vi "Elevator Inline PID.vi"(8 "Manual?":bool, 9 "Setpoint":dbl, 10 "Reset":bool, 11 "Cluster":T10={"Setpoint"=0.0, "Output"=0.0, "DriveMotor"={"DeviceStatus"={"status"=FALSE, "code"=0, "source"=""}, "Type"=enum."PWM", "PWM"={"PWM Channel"=enum."Invalid", "DeadBand"={"Name"="", "maxPositivePwm"=0, "minPositivePwm"=0, "centerPwm"=0, "maxNegativePwm"=0, "minNegativePwm"=0, "angularRange"=0}}, "CAN"={"Device Number"=0, "SetOutput VI Ref"=variant(enum8{"Percent VBus", "Current", "Speed", "Position", "Voltage"} enum."Percent VBus"), "GetOutput VI Ref"=variant(refnum<k1> refnum), "Enable VI Ref"=variant(dbl 12.0), "Disable VI Ref"=variant(enum8{"Percent VBus", "Speed", "Position", "Slave", "Unchanged / Invalid"} enum."Percent VBus"), "Data"=variant(enum16{"Controller 1"} enum."Controller 1")}, "Invert"=FALSE, "DIO PWM"={"PWM \"Enable\" Channel"=enum."Invalid", "DIOChannel"=enum."Invalid", "PWM Rate"=0.0}}, "Encoder"={"DevStatus"={"status"=FALSE, "code"=0, "source"=""}, "EncoderIndex"=enum."Invalid", "CounterIndex"=enum."Invalid", "DistancePerCount"=1.0, "Decoding Type"=enum."4x"}, "notifier"=refnum}) -> (3 "Cluster 2":T10={"Setpoint"=0.0, "Output"=0.0, "DriveMotor"={"DeviceStatus"={"status"=FALSE, "code"=0, "source"=""}, "Type"=enum."PWM", "PWM"={"PWM Channel"=enum."Invalid", "DeadBand"={"Name"="", "maxPositivePwm"=0, "minPositivePwm"=0, "centerPwm"=0, "maxNegativePwm"=0, "minNegativePwm"=0, "angularRange"=0}}, "CAN"={"Device Number"=0, "SetOutput VI Ref"=variant(enum8{"Percent VBus", "Current", "Speed", "Position", "Voltage"} enum."Percent VBus"), "GetOutput VI Ref"=variant(refnum<k1> refnum), "Enable VI Ref"=variant(dbl 12.0), "Disable VI Ref"=variant(enum8{"Percent VBus", "Speed", "Position", "Slave", "Unchanged / Invalid"} enum."Percent VBus"), "Data"=variant(enum16{"Controller 1"} enum."Controller 1")}, "Invert"=FALSE, "DIO PWM"={"PWM \"Enable\" Channel"=enum."Invalid", "DIOChannel"=enum."Invalid", "PWM Rate"=0.0}}, "Encoder"={"DevStatus"={"status"=FALSE, "code"=0, "source"=""}, "EncoderIndex"=enum."Invalid", "CounterIndex"=enum."Invalid", "DistancePerCount"=1.0, "Decoding Type"=enum."4x"}, "notifier"=refnum})   [LabVIEW 2017]
uses:
  <vilib>/Rock Robotics/WPI/MotorControl/WPI_MotorControlDeviceRef.ctl
  <vilib>/Rock Robotics/WPI/MotorControl/WPI_MotorControlType.ctl
  <vilib>/Rock Robotics/SystemInterfaces/DIO/FPGA_DIOPWMChannel.ctl
  <vilib>/Rock Robotics/WPI/PWM/WPI_PWMDeadband.ctl
  <vilib>/Rock Robotics/SystemInterfaces/DIO/FPGA_DIOChannel.ctl
  <vilib>/Rock Robotics/WPI/Encoder/WPI_EncoderDevRef.ctl
  <vilib>/Rock Robotics/SystemInterfaces/Encoder/FPGA_EncoderIdx.ctl
  <vilib>/Rock Robotics/SystemInterfaces/Counter/FPGA_CounterCtrSystemIndex.ctl
  <vilib>/Rock Robotics/WPI/Encoder/WPI_EncoderType.ctl
  Typedef/Controller Message.ctl
  Typedef/FGVAction.ctl
  SimulatorVIs/Simulation Input Global.vi
  <vilib>/ptbypt/NI_PtbyPt.lvlib
panel:
  in  "homing speed":dbl=0.05 format="%#_13g"
  in  "min speed":dbl=0.05 format="%#_13g"
  in  "gravity":dbl=0.003 format="%#_13g"
  in  "PIDF gains":cluster{"Kp":dbl, "Ki":dbl, "Kd":dbl, "Kf":dbl}={"Kp"=0.01, "Ki"=0.0, "Kd"=0.06, "Kf"=0.0} {"Kf" format="%.5f"; "Kd" format="%.3f"; "Ki" format="%.3f"; "Kp" format="%.3f"}
  out "Plant Input":dbl(graph)=0.12000000000000001
  in  "output range":cluster{"output high":dbl, "output low":dbl}={"output high"=1.0, "output low"=-1.0} {"output low" format="%.2f"; "output high" format="%.2f"}
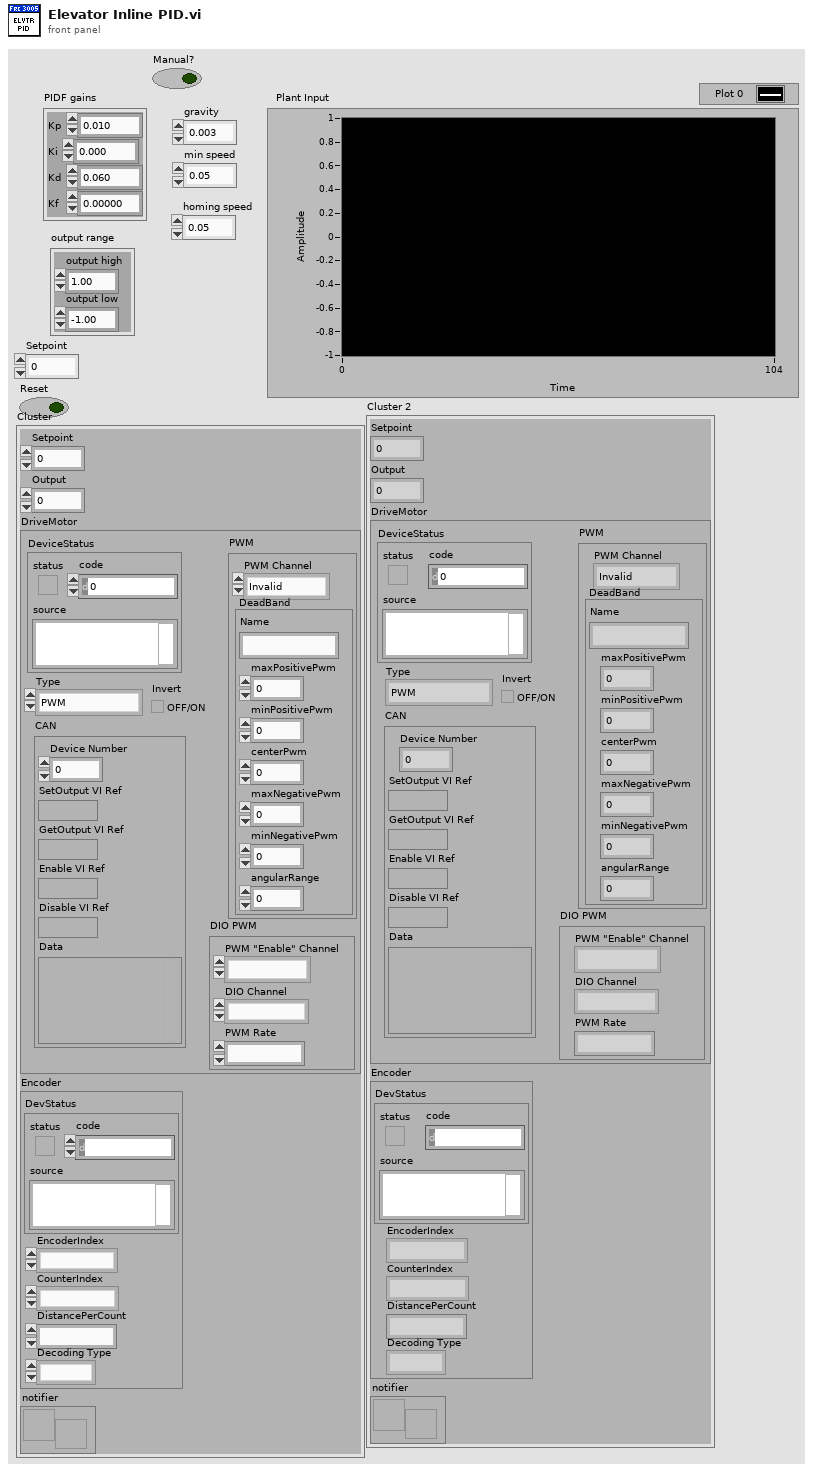
[diagram p1: front panel]
types:
  T1 = typedef "WPI_MotorControlDeviceRef.ctl" = cluster{"DeviceStatus":errorcluster, "Type":T2, "PWM":cluster{"PWM Channel":T3, "DeadBand":T4}, "CAN":cluster{"Device Number":u8, "SetOutput VI Ref":variant, "GetOutput VI Ref":variant, "Enable VI Ref":variant, "Disable VI Ref":variant, "Data":variant}, "Invert":bool, "DIO PWM":cluster{"PWM \"Enable\" Channel":T3, "DIOChannel":T5, "PWM Rate":dbl}}
  T2 = typedef "WPI_MotorControlType.ctl" = enum16{"PWM", "CAN", "DIO PWM"}
  T3 = typedef "FPGA_DIOPWMChannel.ctl" = enum8{"PWM 0", "PWM 1", "PWM 2", "PWM 3", "PWM 4", "PWM 5", "PWM 6", "PWM 7", "PWM 8", "PWM 9", "PWM MXP 0", "PWM MXP 1", "PWM MXP 2", "PWM MXP 3", "PWM MXP 4", "PWM MXP 5", "PWM MXP 6", "PWM MXP 7", "PWM MXP 8", "PWM MXP 9", "Invalid"}
  T4 = typedef "WPI_PWMDeadband.ctl" = cluster{"Name":string, "maxPositivePwm":i32, "minPositivePwm":i32, "centerPwm":i32, "maxNegativePwm":i32, "minNegativePwm":i32, "angularRange":u16}
  T5 = typedef "FPGA_DIOChannel.ctl" = enum8{"DIO 0", "DIO 1", "DIO 2", "DIO 3", "DIO 4", "DIO 5", "DIO 6", "DIO 7", "DIO 8", "DIO 9", "DIO MXP 0", "DIO MXP 1", "DIO MXP 2", "DIO MXP 3", "DIO MXP 4", "DIO MXP 5", "DIO MXP 6", "DIO MXP 7", "DIO MXP 8", "DIO MXP 9", "DIO MXP 10", "DIO MXP 11", "DIO MXP 12", "DIO MXP 13", "DIO MXP 14", "DIO MXP 15", "SPI Port CS1", "SPI Port CS2", "SPI Port CS3", "SPI Port MISO", "SPI Port MOSI", "Invalid"}
  T6 = typedef "WPI_EncoderDevRef.ctl" = cluster{"DevStatus":errorcluster, "EncoderIndex":T7, "CounterIndex":T8, "DistancePerCount":dbl, "Decoding Type":T9}
  T7 = typedef "FPGA_EncoderIdx.ctl" = enum8{"Enc 0", "Enc 1", "Enc 2", "Enc 3", "Enc 4", "Enc 5", "Enc 6", "Enc 7", "Invalid"}
  T8 = typedef "FPGA_CounterCtrSystemIndex.ctl" = enum8{"Ctr 0", "Ctr 1", "Ctr 2", "Ctr 3", "Ctr 4", "Ctr 5", "Ctr 6", "Ctr 7", "Invalid"}
  T9 = typedef "WPI_EncoderType.ctl" = enum16{"1x", "2x", "4x"}
  T10 = cluster{"Setpoint":dbl, "Output":dbl, "DriveMotor":T1, "Encoder":T6, "notifier":refnum<notifier>}
  T11 = typedef "FGVAction.ctl" = enum16{"get", "set"}
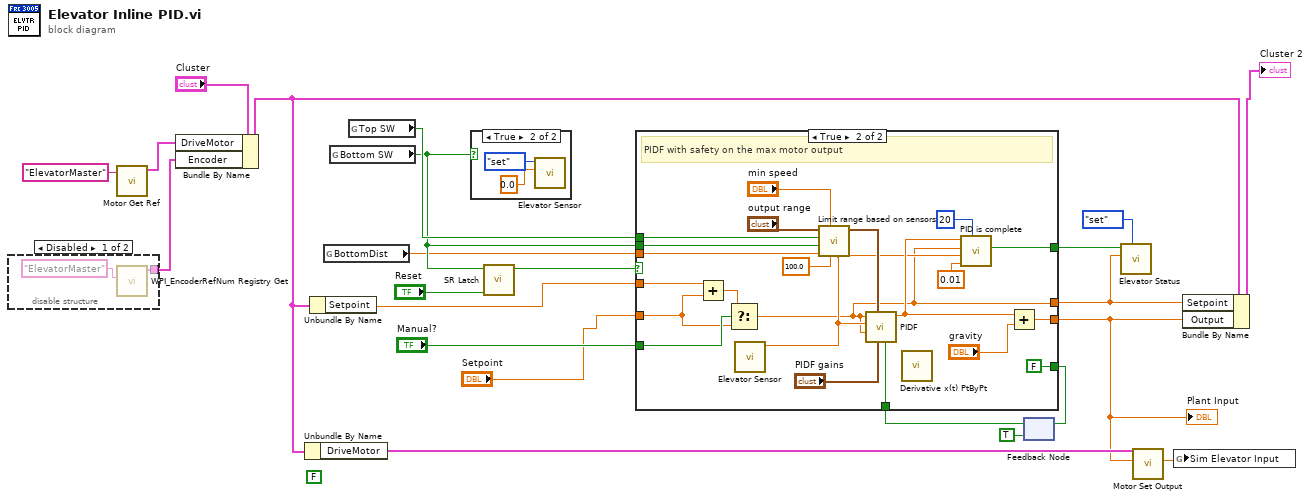
[diagram p0: block diagram]
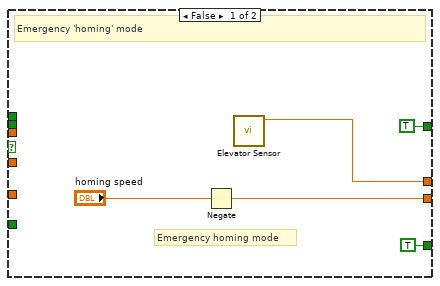
[diagram p2: hidden frame]
diagram:
  (unwired) FALSE
  n1 = disable-structure shown="Disabled" {
    disable-tunnel: [w24 _] -> w19
    frame Disabled {
      n2 = call <vilib>:"WPI_EncoderRefNum Registry Get.vi"("refnum name"="ElevatorMaster") -> ("EncoderDevRef"=w24:T6)  [unwired: 9 in, 1 out]
    }
    frame Enabled {
    }
  }
  n3 = call "Motor Get Ref.vi"("refnum name"="ElevatorMaster") -> ("MotorControlDevRef"=w21:T1)  [unwired: 10 in]
  n4 = Bundle By Name(cluster="Cluster", "DriveMotor"=w21, "Encoder"=w19) -> (w22:T10)
  n5 = Unbundle By Name(w22) -> ("DriveMotor"=w18:T1)
  n6 = Unbundle By Name(w22) -> ("Setpoint"=w6:dbl)
  n7 = global read "Simulation Input Global.vi" "BottomDist"() -> (w13:dbl)
  n8 = global read "Simulation Input Global.vi" "Bottom SW"() -> (w14:bool)
  n9 = global read "Simulation Input Global.vi" "Top SW"() -> (w15:bool)
  n10 = case shown="True" w14 {
    frame False {
    }
    frame True {
      n11 = call "Elevator Sensor.vi"("Value"=0.0, "Action"=FGVAction."set") -> ()  [unwired: 8 in, 2 out]
    }
  }
  n12 = call "SR Latch.vi"("Reset"="Reset", "Value"=w14) -> ("Latched"=w7:bool)  [unwired: 7 in]
  n13 = feedback #1(TRUE ("Reinitialize")) -> (w9:bool)
  n14 = case shown="True" w7 {
    tunnel: "Setpoint" -> [_ w37]
    tunnel: [w30 w49] -> w16
    tunnel: w15 -> [_ w47]
    tunnel: w14 -> [_ w46]
    tunnel: w13 -> [_ w45]
    tunnel: [w29 w33] -> w5
    tunnel: [TRUE ("PID is Done?") w44] -> w11
    tunnel: [TRUE ("Reinitialize") FALSE ("Reinitialize?")] -> w10
    tunnel: w9 -> [_ w43]
    tunnel: "Manual?" -> [_ w41]
    tunnel: w6 -> [_ w39]
    frame False {
      # "Emergency homing mode"
      # "Emergency 'homing' mode"
      n15 = Negate(x="homing speed") -> (-x=w30:dbl)
      n16 = call "Elevator Sensor.vi"() -> ("Value"=w29:dbl)  [unwired: 10 in, 1 out]
    }
    frame True {
      # "PIDF with safety on the max motor output"
      n17 = Add(x=w39, y=w37) -> (x+y=w40:dbl)
      n18 = Select(t=w40, s=w41, f=w37) -> (s? t:f=w33:dbl)
      n19 = call "Elevator Sensor.vi"() -> ("Value"=w35:dbl)  [unwired: 10 in, 1 out]
      n20 = call "Limit range based on sensors.vi"("Position"=w35, "Position Max"=100.0, "min speed"="min speed", "BottomDist"=w45, "Bottom SW"=w46, "Top SW"=w47, "output range in"="output range") -> ("output range out"=w51:cluster{"output high":dbl, "output low":dbl})  [unwired: 4 in]
      n21 = call "PIDF.vi"("reinitialize? (F)"=w43, "PIDF gains"="PIDF gains", "output range"=w51, "Feedforward"=w33, "process variable"=w35, "setpoint"=w33) -> ("output"=w53:dbl)  [unwired: 3 in, 2 out]
      n22 = call <vilib>:"Derivative x(t) PtByPt.vi"() -> ()  [unwired: 4 in, 2 out]
      n23 = call "PID is complete.vi"("sample length"=20, "threshold"=0.01, "process variable"=w35, "setpoint"=w33, "PID Output"=w53) -> ("PID is Done?"=w44:bool)  [unwired: 5 in, 1 out]
      n24 = Add(x=w53, y="gravity") -> (x+y=w49:dbl)
    }
  }
  "Plant Input" <- w16
  n25 = feedback-in #1(w10) -> ()
  n26 = call "Elevator Status.vi"("Action"=FGVAction."set", "SP in"=w5, "Moving? (F)"=w11) -> ()  [unwired: 6 in, 3 out]
  n27 = call "Motor Set Output.vi"("output"=w16, "DriveMotor"=w18) -> ("Motor Output"=w17:dbl)  [unwired: 9 in]
  n28 = global write "Simulation Input Global.vi" "Sim Elevator Input"(w17) -> ()
  n29 = Bundle By Name(cluster=w22, "Setpoint"=w5, "Output"=w16) -> (→"Cluster 2":T10)
